vi "Sort Shots.vi"(1 "shot array":T1[](array[typedef]) {"UncorrectedAvgVel_PB" format="%.1f"; "strikeVel_PB" format="%.1f"; "velLoss_PB" format="%.1f"; "avgVel_PB" format="%.1f"; "Redundant_Velocity" format="%.1f"; "Energy Loss (J)" format="%.3e"; "Projectile Mass" min=0 step=1 format="%.4f"; "Corrected residual" format="%.2f"; "Uncorrected Residual" format="%.2f"; "Corrected Impact" format="%.2f"; "Uncorrected Impact" format="%.2f"; "Shot Angle" max=90 step=1; "SHOT STATUS" items=["Partial", "Complete"]; "IMPACT VELOCITY" min=0 max=10000 step=0.1 format="%.1f"; "Barrel Temperature" format="%.1f"; "Powder Loading" format="%.4f"; "RESIDUAL  VELOCITY" min=0 max=10000 step=0.1 format="%.1f"}) -> (0 "shotTable OUT":string[][](array[string]))   [LabVIEW 2012]
uses:
  Shot Record.ctl
panel:
  # "Order"
  # "Chrono#1"
  # "Chrono#2"
  # "Average"
  # "Vel Loss"
  # "Strike Vel"
  # "Residual"
  # "Status"
  # "Depth"
  # "Diameter"
  # "Loading"
  # "Description"
  # "Order"
  # "Chrono#1"
  # "Loading"
  # "Status"
  # "Residual"
  # "Depth"
  # "Diameter"
  # "Description"
  # "Chrono#2"
  # "Average"
  # "Vel Loss"
  # "Strike Vel"
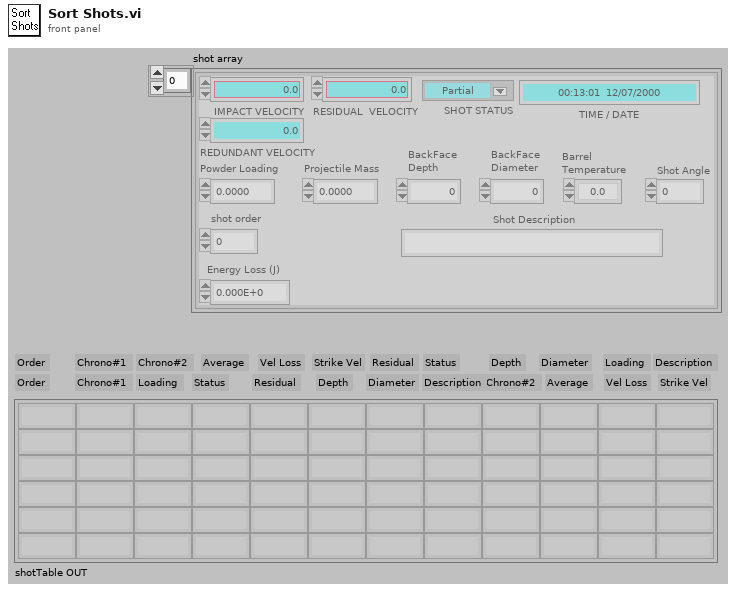
[diagram p1: front panel]
types:
  T1 = typedef "Shot Record.ctl" = cluster{"avgVel_PB":sgl, "IMPACT VELOCITY":sgl, "RESIDUAL  VELOCITY ":sgl, "Shot Description":string, "Powder Loading ":sgl, "Barrel Temperature":sgl, "TIME / DATE":string, "shot order":i32, "SHOT STATUS":u16, "Shot Angle":u16, "Uncorrected Impact":sgl, "Corrected Impact":sgl, "Uncorrected Residual":sgl, "Corrected residual":sgl, "Projectile Mass":sgl, "usedv50":bool, "Energy Loss (J)":sgl, "BackFace\nDepth":sgl, "BackFace\nDiameter":sgl, "Redundant_Velocity":sgl, "velLoss_PB":sgl, "strikeVel_PB":sgl, "UncorrectedRed_PB":sgl, "CorrectedRed_PB":sgl, "UncorrectedAvgVel_PB":sgl}
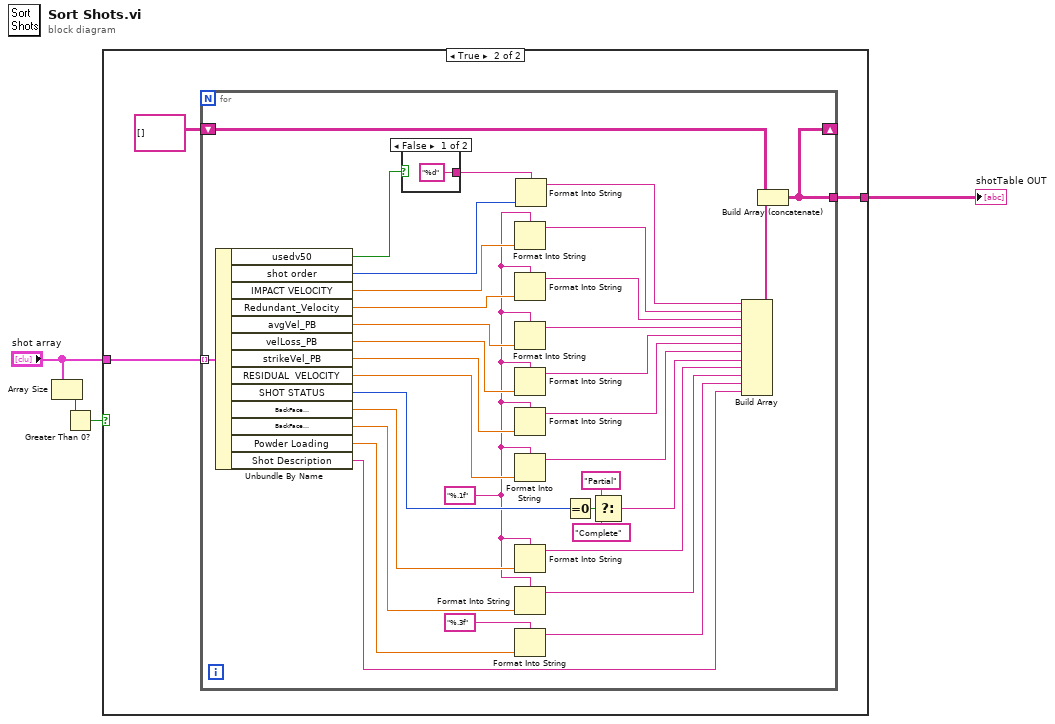
[diagram p0: block diagram]
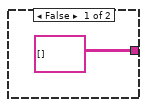
[diagram p2: hidden frame]
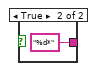
[diagram p3: hidden frame]
diagram:
  n1 = Array Size(array="shot array") -> (size(s)=w4:i32)
  n2 = Greater Than 0?(x=w4) -> (x > 0?=w1:bool)
  n3 = case shown="True" w1 {
    tunnel: "shot array" -> [_ w6]
    tunnel: [string[][] [] w7] -> w2
    frame False {
    }
    frame True {
      n4 = for {
        tunnel: w6 -> [w30] mode=indexing
        shift-right: [w38] -> _
        shift-left: string[][] [] -> [w42]
        tunnel: [w38] -> w7
        w9 = "%.1f" ("Format String")
        n5 = Unbundle By Name(w30) -> ("usedv50"=w29:bool, "shot order"=w28:i32, "IMPACT VELOCITY"=w27:sgl, "Redundant_Velocity"=w26:sgl, "avgVel_PB"=w25:sgl, "velLoss_PB"=w24:sgl, "strikeVel_PB"=w23:sgl, "RESIDUAL  VELOCITY"=w17:sgl, "SHOT STATUS"=w13:u16, "BackFace\nDepth"=w22:sgl, "BackFace\nDiameter"=w21:sgl, "Powder Loading"=w20:sgl, "Shot Description"=w19:string)
        n6 = case shown="False" w29 {
          tunnel: ["%d" "%d*"] -> w37
          frame False {
          }
          frame True {
          }
        }
        n7 = Format Into String(format string=w9, w27) -> (resulting string=w39:string)  [unwired: 2 in, 1 out]
        n8 = Format Into String(format string=w9, w26) -> (resulting string=w40:string)  [unwired: 2 in, 1 out]
        n9 = Format Into String(format string=w9, w25) -> (resulting string=w18:string)  [unwired: 2 in, 1 out]
        n10 = Format Into String(format string=w9, w24) -> (resulting string=w35:string)  [unwired: 2 in, 1 out]
        n11 = Format Into String(format string=w9, w23) -> (resulting string=w34:string)  [unwired: 2 in, 1 out]
        n12 = Format Into String(format string=w9, w17) -> (resulting string=w11:string)  [unwired: 2 in, 1 out]
        n13 = Format Into String(format string=w9, w22) -> (resulting string=w33:string)  [unwired: 2 in, 1 out]
        n14 = Format Into String(format string=w9, w21) -> (resulting string=w32:string)  [unwired: 2 in, 1 out]
        n15 = Format Into String(format string="%.3f" ("Format String"), w20) -> (resulting string=w31:string)  [unwired: 2 in, 1 out]
        n16 = Format Into String(format string=w37, w28) -> (resulting string=w36:string)  [unwired: 2 in, 1 out]
        n17 = Equal To 0?(x=w13) -> (x = 0?=w14:bool)
        n18 = Select(t="Partial", s=w14, f="Complete") -> (s? t:f=w12:string)
        n19 = Build Array(w36, w39, w40, w18, w35, w34, w11, w12, w33, w32, w31, w19) -> (w41:string[])
        n20 = Build Array (concatenate)(w42, w41) -> (w38:string[][])
      }
    }
  }
  "shotTable OUT" <- w2
